vi "Read.vi"(8 "error in (no error)":errorcluster, 10 "Timeout":i32, 11 "DataShare in":refnum<class "DataShare.lvclass">) -> (0 "error out":errorcluster, 1 "Timed Out?":bool, 2 "Data":variant, 3 "DataShare out":refnum<class "DataShare.lvclass">)   [LabVIEW 2014, in "DataShare.lvclass"]
uses:
  DataShare.lvclass
  DataShare.lvclass/DataShare.ctl
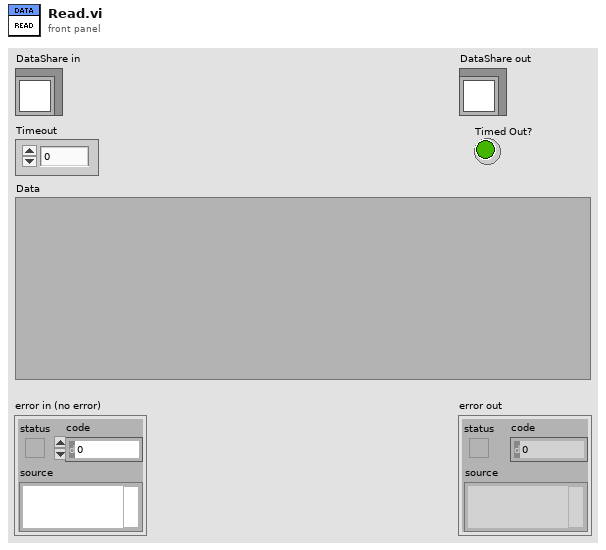
[diagram p1: front panel]
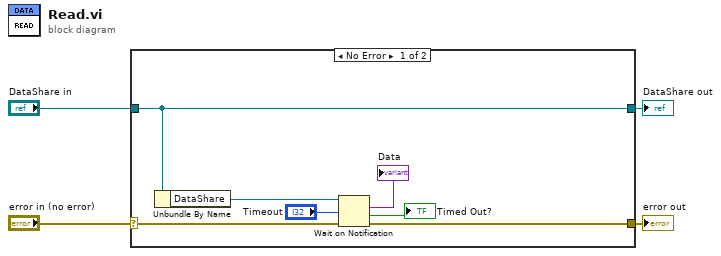
[diagram p0: block diagram]
diagram:
  n1 = case shown="No Error" "error in (no error)" {
    selector: "error in (no error)" -> [w8 w13]
    tunnel: [w7 w13] -> w3
    tunnel: [w11 w12] -> w1
    tunnel: "DataShare in" -> [w11 w12]
    frame No Error {
      n2 = Unbundle By Name(w11) -> ("DataShare"=w10:refnum<notifier>)
      n3 = Wait on Notification(notifier=w10, timeout in ms (-1)="Timeout", error in (no error)=w8) -> (notification=→"Data":variant, timed out?=→"Timed Out?":bool, error out=w7:errorcluster)  [unwired: 1 in, 1 out]
    }
    frame Error {
    }
  }
  "error out" <- w3
  "DataShare out" <- w1
